vi "Ramsete_Execute.vi"(4 "Enabled":bool=TRUE, 6 "Reset":bool, 7 "RAMSETE_EXE_TUNING":T4={"B"=2.0, "Zeta"=0.7, "X Tolerance M"=2.0, "Y Tolerance M"=0.7, "Heading Tolerance RAD"=0.7, "Track Width M"=2.0, "Max Speed M/S"=2.0} {"Max Speed M/S" format="%13.4f"; "Track Width M" format="%13.4f"; "Heading Tolerance RAD" format="%13.4f"; "Y Tolerance M" format="%13.4f"; "X Tolerance M" format="%13.4f"; "Zeta" format="%13.4f"; "B" format="%13.4f"}, 8 "Gyro-Radians\n(Inc counterclockwise)":dbl, 9 "RightDist-Meters":dbl, 10 "LeftDist-Meters":dbl, 11 "TRAJ_STATE":T6 {"POSE"."ROTATION"."SIN" format="%13.4f"; "POSE"."ROTATION"."COS" format="%13.4f"; "POSE"."ROTATION"."VALUE" format="%13.4f"; "POSE"."TRANSLATION"."Y" format="%14.3f"; "POSE"."TRANSLATION"."X" format="%14.3f"}) -> (0 "CurrentRelativePose":T1 {"ROTATION"."SIN" format="%13.4f"; "ROTATION"."COS" format="%13.4f"; "ROTATION"."VALUE" format="%13.4f"; "TRANSLATION"."Y" format="%14.3f"; "TRANSLATION"."X" format="%14.3f"}, 1 "AtReference":bool, 2 "Right Speed Dmd M/S":dbl, 3 "Left Speed Dmd M/S":dbl, 5 "outRAMSETE":T5={"B"=2.0, "Zeta"=0.7, "poseTolerance"={"TRANSLATION"={"X"=0.0, "Y"=0.0}, "ROTATION"={"VALUE"=0.0, "COS"=1.0, "SIN"=0.0}}, "poseError"={"TRANSLATION"={"X"=0.0, "Y"=0.0}, "ROTATION"={"VALUE"=0.0, "COS"=1.0, "SIN"=0.0}}, "Enabled"=TRUE} {"poseError"."ROTATION"."SIN" format="%13.4f"; "poseError"."ROTATION"."COS" format="%13.4f"; "poseError"."ROTATION"."VALUE" format="%13.4f"; "poseError"."TRANSLATION"."Y" format="%14.3f"; "poseError"."TRANSLATION"."X" format="%14.3f"; "poseTolerance"."ROTATION"."SIN" format="%13.4f"; "poseTolerance"."ROTATION"."COS" format="%13.4f"; "poseTolerance"."ROTATION"."VALUE" format="%13.4f"; "poseTolerance"."TRANSLATION"."Y" format="%14.3f"; "poseTolerance"."TRANSLATION"."X" format="%14.3f"; "Zeta" format="%12.3f"; "B" format="%12.3f"})   [LabVIEW 2019, in "Trajectory_Library.lvlib"]
doc: "Convienience function to create and calculate the ramsete control, returning normalized desired left and right speed setpoints \n\n\nParameters: \n - Ramsete EXE Tuning -- Packed data cluster containing the ramsete tuning parameters and Differntial Drive kinematics information.\n - TrajState - Desired trajectory state\n - Left Dist -- The left distance read from encoders (Meters). The encoders do NOT have to be reset at the beginning of trajectory execution.\n - Right Dist -- The right distance read from encoders (Meters). The encoders do NOT have to be reset at the beginning of trajectory execution.\n - Gyro - The current reading of a gyro whose value increases counter clockwise. (You may need to negate your gyro reading.) (Radians)\n - Reset -- Resets the current robot pose and the beginning left and right distances and the gyro reading\n - Enabled -- When enabled uses the ramsete closed loop control to drive the left and right speed demand outputs. When disabled the trajectory data is directly converted to left and right speed demands.\n\n\nReturns:\n - Left Speed Dmd -- Left Speed demand (Meters/Second)\n - Right Speed Dmd -- Right Speed demand (Meters/Second)\n - Out Ramsete -- Updated Ramsete data structure\n - Current Relative Pose -- Current robot relative pose. This pose is reset to zero when the RESET input is set to TRUE. \n - At Reference -- Set to TRUE when the current robot pose is withing the specified tolerance of the desired POSE from the trajectory state input."
uses:
  Trajectory_Library.lvlib
  TRAJ_STATE.ctl
  POSE2D.ctl
  TRANSLATION2D.ctl
  ROTATION2D.ctl
  RAMSETE.ctl
  RAMSETE_EXE_TUNING.ctl
  Rotation_CreateAngle.vi
  Translation_Create.vi
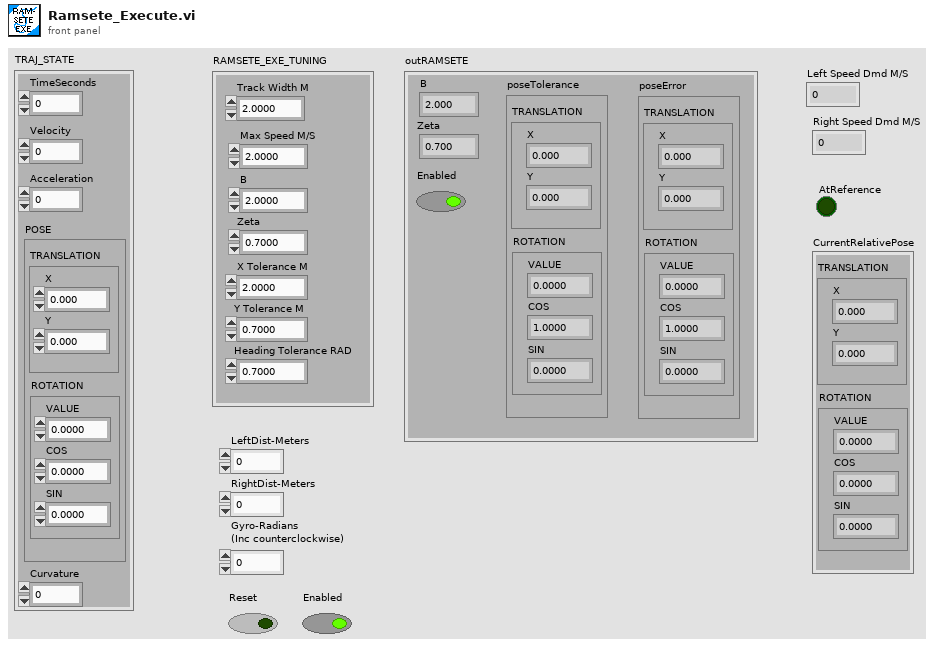
[diagram p1: front panel]
types:
  T1 = typedef "Trajectory_Library.lvlib/POSE2D.ctl" = cluster{"TRANSLATION":T2, "ROTATION":T3}
  T2 = typedef "Trajectory_Library.lvlib/TRANSLATION2D.ctl" = cluster{"X":dbl, "Y":dbl}
  T3 = typedef "Trajectory_Library.lvlib/ROTATION2D.ctl" = cluster{"VALUE":dbl, "COS":dbl, "SIN":dbl}
  T4 = typedef "Trajectory_Library.lvlib/RAMSETE_EXE_TUNING.ctl" = cluster{"B":dbl, "Zeta":dbl, "X Tolerance M":dbl, "Y Tolerance M":dbl, "Heading Tolerance RAD":dbl, "Track Width M":dbl, "Max Speed M/S":dbl}
  T5 = typedef "Trajectory_Library.lvlib/RAMSETE.ctl" = cluster{"B":dbl, "Zeta":dbl, "poseTolerance":T1, "poseError":T1, "Enabled":bool}
  T6 = typedef "Trajectory_Library.lvlib/TRAJ_STATE.ctl" = cluster{"TimeSeconds":dbl, "Velocity":dbl, "Acceleration":dbl, "POSE":T1, "Curvature":dbl}
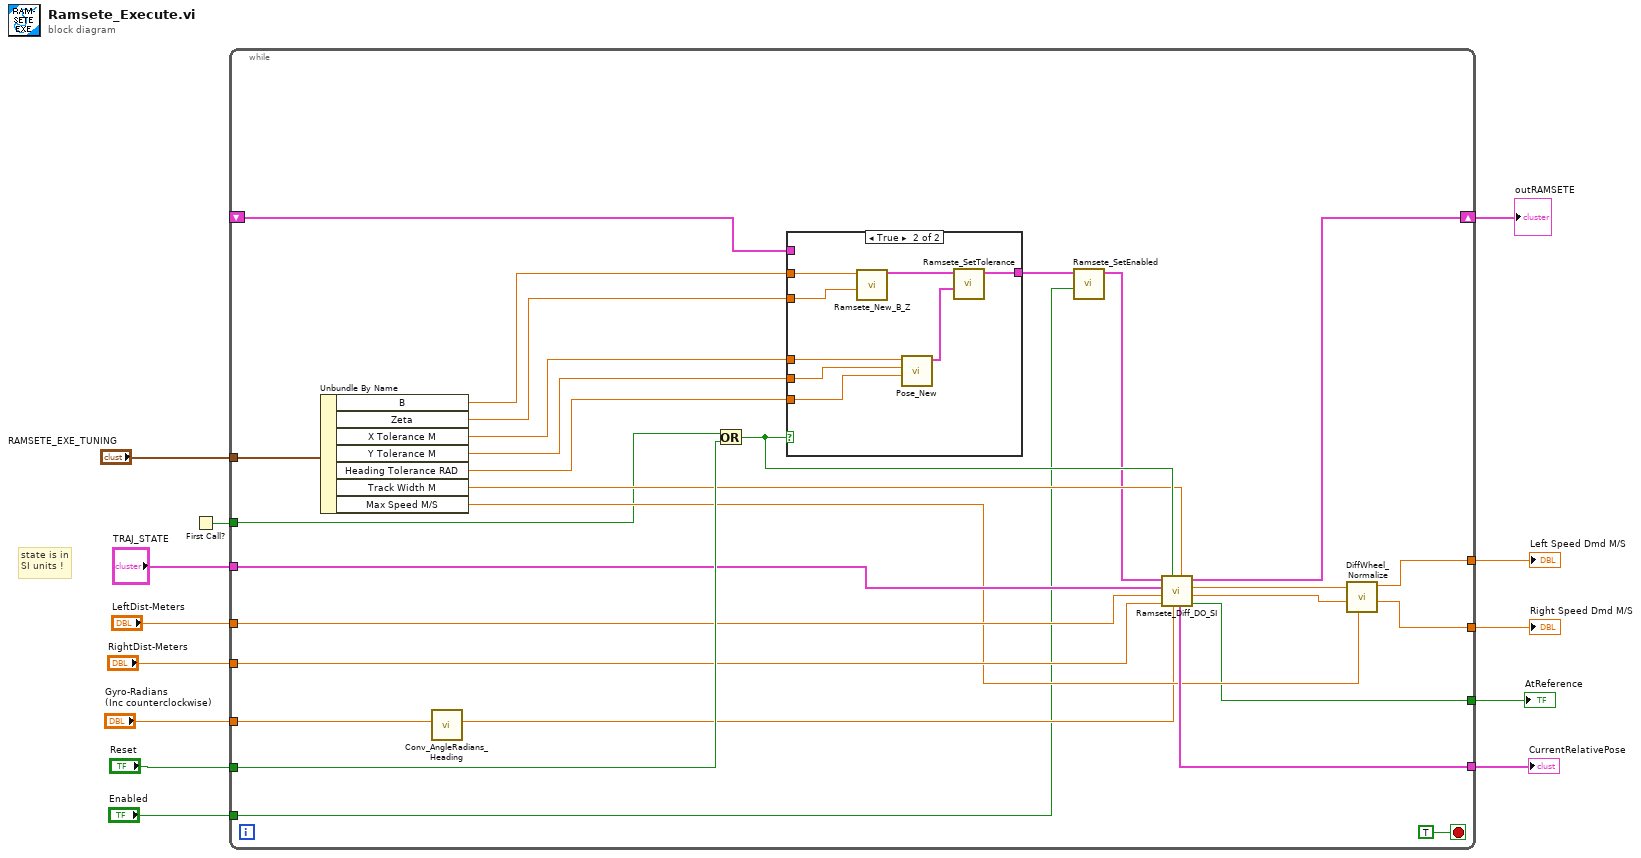
[diagram p0: block diagram]
diagram:
  # "state is in\nSI units !"
  n1 = First Call?() -> (First Call?: T/F=w1:bool)
  n2 = while {
    tunnel: "RAMSETE_EXE_TUNING" -> [w41]
    tunnel: "TRAJ_STATE" -> [w31]
    tunnel: "LeftDist-Meters" -> [w30]
    tunnel: "RightDist-Meters" -> [w29]
    tunnel: [w28] -> w7
    tunnel: [w24] -> w6
    tunnel: [w23] -> w5
    tunnel: "Gyro-Radians\n(Inc counterclockwise)" -> [w21]
    tunnel: "Enabled" -> [w17]
    tunnel: "Reset" -> [w40]
    tunnel: [w22] -> w4
    tunnel: w1 -> [w16]
    shift-right: [w34] -> w11
    shift-left: _ -> [w15]
    stop <- TRUE stop-if-true
    n3 = Unbundle By Name(w41) -> ("B"=w39:dbl, "Zeta"=w38:dbl, "X Tolerance M"=w37:dbl, "Y Tolerance M"=w36:dbl, "Heading Tolerance RAD"=w35:dbl, "Track Width M"=w32:dbl, "Max Speed M/S"=w25:dbl)
    n4 = call "Conv_AngleRadians_Heading.vi"("Radians"=w21) -> ("Heading"=w20:dbl)  [unwired: 10 in]
    n5 = Or(x=w16, y=w40) -> (x .or. y?=w33:bool)
    n6 = case shown="True" w33 {
      tunnel: w39 -> [_ w50]
      tunnel: w38 -> [_ w49]
      tunnel: w37 -> [_ w46]
      tunnel: w36 -> [_ w45]
      tunnel: w35 -> [_ w44]
      tunnel: [w42 w43] -> w19
      tunnel: w15 -> [w42 _]
      frame False {
      }
      frame True {
        n7 = call "Ramsete_New_B_Z.vi"("Zeta"=w49, "B"=w50) -> ("outRAMSETE"=w48:T5)  [unwired: 9 in]
        n8 = call "Pose_New.vi"("Heading"=w44, "Y"=w45, "X"=w46) -> ("out POSe"=w47:T1)  [unwired: 8 in]
        n9 = call "Ramsete_SetTolerance.vi"("tolerancePose"=w47, "inRAMSETE"=w48) -> ("outRAMSETE"=w43:T5)  [unwired: 9 in]
      }
    }
    n10 = call "Ramsete_SetEnabled.vi"("Enabled"=w17, "inRAMSETE"=w19) -> ("outRAMSETE"=w18:T5)  [unwired: 9 in]
    n11 = call "Ramsete_Diff_DO_SI.vi"("WheelBase-Meters"=w32, "Gyro-Radians"=w20, "Reset"=w33, "RightDist-Meters"=w29, "LeftDist-Meters"=w30, "TRAJ_STATE"=w31, "inRAMSETE"=w18) -> ("AtReference"=w22:bool, "RightVelDmd"=w26:dbl, "LeftVelDmd"=w27:dbl, "outRAMSETE"=w34:T5, "CurrentRelativePose"=w28:T1)
    n12 = call "DiffWheel_Normalize.vi"("Max Speed"=w25, "Right Wheel Demand"=w26, "Left Wheel Demand"=w27) -> ("Normalized Right Wheel Demand"=w23:dbl, "Normalized Left Wheel Demand"=w24:dbl)  [unwired: 7 in]
  }
  "outRAMSETE" <- w11
  "CurrentRelativePose" <- w7
  "Left Speed Dmd M/S" <- w6
  "Right Speed Dmd M/S" <- w5
  "AtReference" <- w4
